vi "TTA_MATLAB_RFIC_PALLinearization_DetailedResults.vi"(8 "error in":errorcluster, 10 "TestGroup":string, 11 "SubTest":string) -> (0 "error out":errorcluster, 3 "SubTestSuccess":dbl[](array[numeric]))   [LabVIEW 2016]
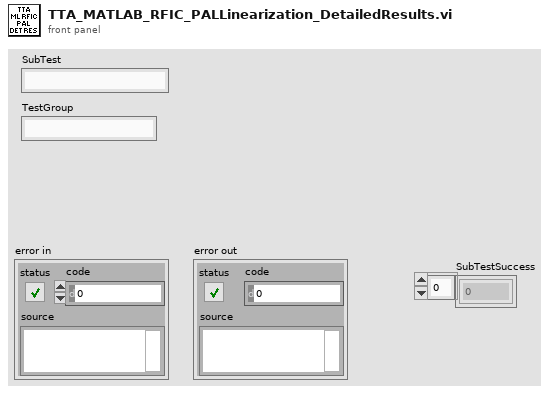
[diagram p1: front panel]
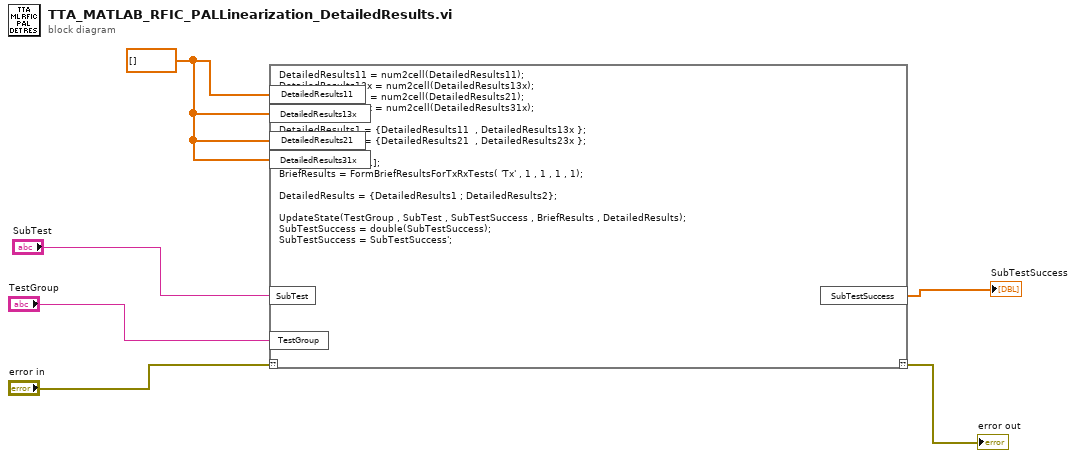
[diagram p0: block diagram]
diagram:
  w1 = dbl[] []
  n1 = script code="DetailedResults11 = num2cell(DetailedResults11);\nDetailedResults13x = num2cell(DetailedResults13x);\nDetailedResults21 = num2cell(DetailedResults21);\nDetailedResults31x = num2cell(DetailedResults31x);\n\nDetailedResults1 = {DetailedResults11  , DetailedResults13x };\nDetailedResults2 = {DetailedResults21  , DetailedResults23x };\n\nSuccessList = [1 ; 1];\nBriefResults = FormBriefResultsForTxRxTests( 'Tx' , 1 , 1 , 1 , 1);\n                                            \nDetailedResults = {DetailedResults1 ; DetailedResults2};\n\nUpdateState(TestGroup , SubTest , SubTestSuccess , BriefResults , DetailedResults);\nSubTestSuccess = double(SubTestSuccess);\nSubTestSuccess = SubTestSuccess';"("??"="error in", "SubTest"="SubTest", "TestGroup"="TestGroup", "DetailedResults11"=w1, "DetailedResults13x"=w1, "DetailedResults21"=w1, "DetailedResults31x"=w1) -> ("??"=→"error out":errorcluster, "SubTestSuccess"=→"SubTestSuccess":dbl[])
